vi "FGV_in_file.vi"(2 "data":string) -> (7 "data":string)   [LabVIEW 2015]
uses:
  ref_tools/polys/poly_this_vis_path.vi
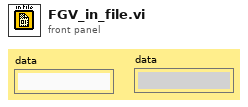
[diagram p1: front panel]
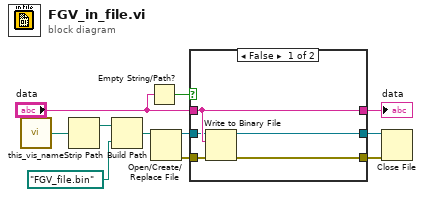
[diagram p0: block diagram]
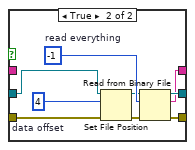
[diagram p2: hidden frame]
diagram:
  n1 = call-poly "this_vis_name.vi"() -> ("your path"=w6:path)  [unwired: 9 in]
  n2 = Strip Path(path=w6) -> (stripped path=w5:path)  [unwired: 1 out]
  n3 = Build Path(base path=w5, name or relative path=path "FGV_file.bin" ("path to cache")) -> (appended path=w3:path)
  n4 = Empty String/Path?(string/path="data") -> (empty?=w7:bool)
  n5 = Open/Create/Replace File(file path (use dialog)=w3) -> (refnum out=w2:refnum<file>, error out=w1:errorcluster)  [unwired: 5 in, 1 out]
  n6 = case shown="False" w7 {
    tunnel: "data" -> [w14 _]
    tunnel: [w14 w23] -> w9
    tunnel: [w16 w25] -> w11
    tunnel: [w15 w24] -> w10
    tunnel: w2 -> [w13 w18]
    tunnel: w1 -> [w12 w17]
    frame False {
      n7 = Write to Binary File(file (use dialog)=w13, data=w14, error in=w12) -> (refnum out=w15:refnum<file>, error out=w16:errorcluster)  [unwired: 3 in, 1 out]
    }
    frame True {
      w21 = i64 4  # data offset
      w22 = -1  # read everything
      n8 = Set File Position(offset (in bytes) (0)=w21, refnum=w18, error in=w17) -> (refnum out=w20:refnum<file>, error out=w19:errorcluster)  [unwired: 1 in]
      n9 = Read from Binary File(8:w19, 10:w22, 11:w20) -> (0:w25:errorcluster, 2:w23:string, 3:w24:refnum<file>)  [unwired: 3 in, 1 out]
    }
  }
  "data" <- w9
  n10 = Close File(refnum=w10, error in=w11) -> ()  [unwired: 2 out]
